vi "GUILib.simple numeric update.vi"(0 "ctlRef":refnum<vi>, 1 "isNominal":bool, 2 "value":dbl=nan, 4 "valueStatus":T1, 5 "error in (no error)":errorcluster) -> (14 "ctlRef dup":refnum<vi>, 19 "error out":errorcluster)   [LabVIEW 2012, in "GUILib.lvlib"]
doc: "updates a value for a specific type of control"
uses:
  GUILib.lvlib
  UtilityLib/UtilityLib.valueStatus.ctl
  UtilityLib/UtilityLib.lvlib
panel:
  in  "numericType":dbl step=22.0
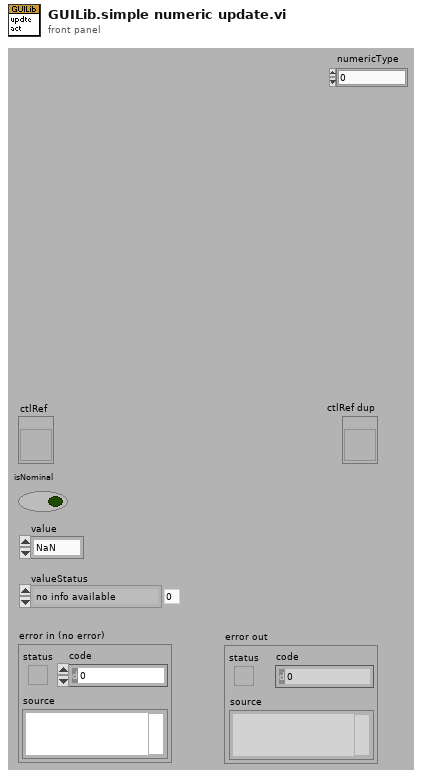
[diagram p1: front panel]
types:
  T1 = typedef "UtilityLib.lvlib/UtilityLib.valueStatus.ctl" = enum16{"no info available", "stand by/off", "on", "warning", "alarm/malfunction", "not implemented", "user action required", "important information", "system default", "control default", "indicator default", "button default"}
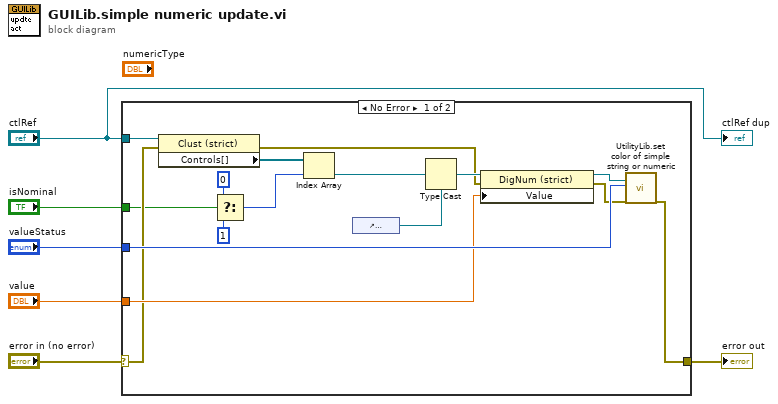
[diagram p0: block diagram]
diagram:
  n1 = case shown="No Error" "error in (no error)" {
    selector: "error in (no error)" -> [w14 w23]
    tunnel: "ctlRef" -> [w19 _]
    tunnel: "valueStatus" -> [w18 _]
    tunnel: "value" -> [w16 _]
    tunnel: [w11 w23] -> w3
    tunnel: "isNominal" -> [w10 _]
    frame No Error {
      n2 = property on="Property Node" class="Clust (strict)"(reference=w19, error in=w14) -> (error out=w13:errorcluster, "Controls[]"=w20:refnum<vi>[])  [unwired: 1 out]
      n3 = Select(t=0, s=w10, f=1 ("index")) -> (s? t:f=w7:i32)
      n4 = Index Array(array=w20, index=w7) -> (element=w21:refnum<vi>)
      n5 = control-ref of="numericType"() -> (w22:refnum<vi>)
      n6 = Type Cast(type=w22, x=w21) -> (*(type *) &x=w17:refnum<vi>)
      n7 = property on="Property Node" class="DigNum (strict)"(reference=w17, error in=w13, "Value"=w16) -> (reference out=w15:refnum<vi>, error out=w12:errorcluster)
      n8 = call "UtilityLib.set color of simple string or numeric.vi"("simpleNumeric"=w15, "valueStatus"=w18, "error in (no error)"=w12) -> ("error out"=w11:errorcluster)  [unwired: 16 in]
    }
    frame Error {
    }
  }
  "error out" <- w3
  "ctlRef dup" <- "ctlRef"
